vi "qDIP.vi"(0 "System no.":i32=1 min=1 max=4 step=1, 2 "DI's to query":string[](array[string]), 3 "All DI's?":bool, 4 "DI identifier?":bool=TRUE, 5 "error in":errorcluster) -> (14 "Pulse detected?":bool[](array[boolean]), 19 "error out":errorcluster)   [LabVIEW 2020]
doc: "Returns if a digital pulse was detected since last call of DIP?.\n\nE-816: If All DI's = TRUE, then DI identifier can be FALSE. DI's to query are 1. Check controller manual to find out if DIP? is supported."
panel:
  # "Returns if a digital pulse was detected since last call of DIP?."
  # "Query"
  # "If all DI's:"
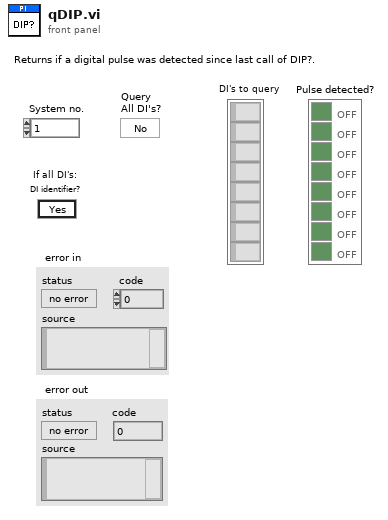
[diagram p1: front panel]
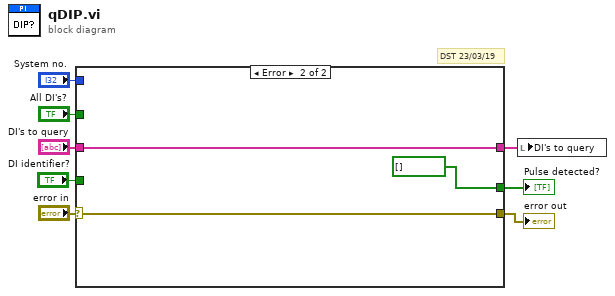
[diagram p0: block diagram]
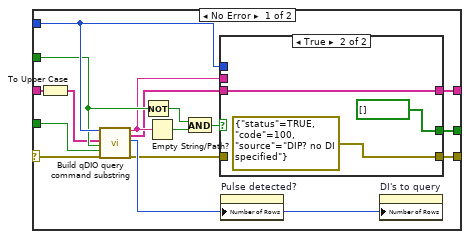
[diagram p2: hidden frame]
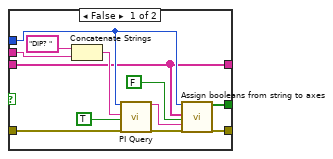
[diagram p3: hidden frame]
diagram:
  # "DST 23/03/19"
  n1 = case shown="Error" "error in" {
    selector: "error in" -> [w9 w41]
    tunnel: [w15 bool[] [] ("Booleans")] -> w8
    tunnel: "DI's to query" -> [w24 w40]
    tunnel: [w23 w41] -> w6
    tunnel: "DI identifier?" -> [w22 _]
    tunnel: "System no." -> [w21 _]
    tunnel: "All DI's?" -> [w16 _]
    tunnel: [w10 w40] -> w2
    frame No Error {
      n2 = To Upper Case(1:w24) -> (0:w14:string[])
      n3 = call "Build qDIO query command substring.vi"("System no."=w21, "DI's to query in"=w14, "Query all DI's?"=w16, "For all DI's: use\nDI identifier?"=w22, "error in"=w9) -> ("Command substring"=w13:string, "DI's to query out"=w11:string[], "Number of rows"=w18:u32, "error out"=w17:errorcluster)  [unwired: 1 in, 10 out]
      n4 = Not(x=w16) -> (.not. x?=w19:bool)
      n5 = Empty String/Path?(string/path=w13) -> (empty?=w20:bool)
      n6 = And(x=w19, y=w20) -> (x .and. y?=w12:bool)
      n7 = case shown="True" w12 {
        tunnel: [w28 errorcluster {"status"=TRUE, "code"=100, "source"="DIP? no DI specified"} ("error out")] -> w23
        tunnel: w21 -> [w33 _]
        tunnel: w17 -> [w32 _]
        tunnel: [w31 bool[] [] ("Booleans")] -> w15
        tunnel: w13 -> [w29 _]
        tunnel: w11 -> [w27 w37]
        tunnel: [w27 w37] -> w10
        frame False {
          n8 = Concatenate Strings("DIP? ", w29) -> (w34:string)
          n9 = call "PI Query.vi"("System no."=w33, "String to send"=w34, "Attach termination char.?"=TRUE ("Attach Linefeed?"), "error in"=w32) -> ("String read"=w26:string, "error out"=w25:errorcluster)  [unwired: 3 in, 11 out]
          n10 = call "Assign booleans from string to axes.vi"("System no."=w33, "Queried axes"=w27, "All axes queried?"=FALSE, "Input String"=w26, "error in"=w25) -> ("Booleans"=w31:bool[], "error out"=w28:errorcluster)  [unwired: 13 out]
        }
        frame True {
        }
      }
      n11 = property on="Pulse detected?" class="Arr (strict)"("Number of Rows"=w18) -> ()  [unwired: 2 in, 2 out]
      n12 = property on="DI's to query" class="Arr (strict)"("Number of Rows"=w18) -> ()  [unwired: 2 in, 2 out]
    }
    frame Error {
    }
  }
  "error out" <- w6
  "Pulse detected?" <- w8
  n13 = local write "DI's to query"(w2) -> ()
